vi "Ignore-error.vi"   [LabVIEW 2013, in "SLMControl.lvlib" / "SC-Main.lvclass"]
uses:
  SC-Main.lvclass
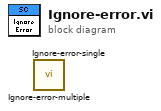
[diagram p0: block diagram]
diagram:
  n1 = call "Ignore-error-multiple.vi"() -> ()  [unwired: 11 in, 1 out]
  n2 = call "Ignore-error-single.vi"() -> ()  [unwired: 11 in, 1 out]
